vi "Show Hide (Label).vi"(5 "Invert? [F]":bool, 7 "Regex? [F]":bool, 8 "error in (no error)":errorcluster, 9 "Show? [T]":bool=TRUE, 10 "Label":string, 11 "MMI Scaling in":refnum<class "Alternative.lvclass">) -> (0 "error out":errorcluster, 2 "Match?":bool, 3 "MMI Scaling out":refnum<class "Alternative.lvclass">)   [LabVIEW 2021, in "Alternative.lvclass"]
doc: "Copyright 2018, Wiebe Walstra, wiebe@carya.nl."
uses:
  Alternative.lvclass
  C:/Projects/Dynamic-Scaling/Dynamic Scaling/IContainer/IContainer.lvclass
  IContainer.lvclass
  IObject.lvclass
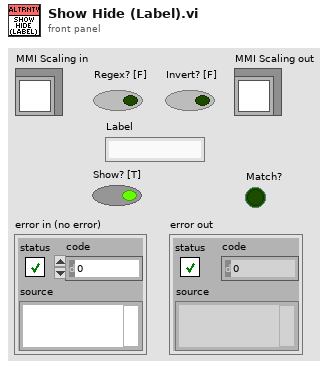
[diagram p1: front panel]
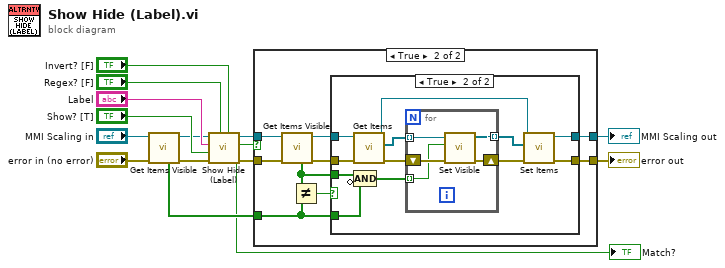
[diagram p0: block diagram]
diagram:
  n1 = call "Get Items Visible.vi"("error in (no error)"="error in (no error)", "IContainer in"="MMI Scaling in") -> ("error out"=w4:errorcluster, "IContainer out"=w7:refnum<class "Alternative.lvclass">, "Items visible"=w2:bool[])  [unwired: 6 in, 1 out]
  n2 = call-parent "Show Hide (Label).vi"("Invert? [F]"="Invert? [F]", "Regex? [F]"="Regex? [F]", "error in (no error)"=w4, "Show? [T]"="Show? [T]", "Label"="Label", "MMI Scaling in"=w7) -> ("error out"=w14:errorcluster, "Match?"=w1:bool, "MMI Scaling out"=w3:refnum<class "Alternative.lvclass">)  [unwired: 3 in]
  "Match?" <- w1
  n3 = case shown="True" w1 {
    tunnel: w14 -> [w15 w25]
    tunnel: [w15 w24] -> w9
    tunnel: [w16 w23] -> w8
    tunnel: w3 -> [w16 w21]
    tunnel: w2 -> [_ w18]
    frame False {
    }
    frame True {
      n4 = call "Get Items Visible.vi"("error in (no error)"=w25, "IContainer in"=w21) -> ("error out"=w22:errorcluster, "IContainer out"=w20:refnum<class "Alternative.lvclass">, "Items visible"=w19:bool[])  [unwired: 6 in, 1 out]
      n5 = Not Equal?(x=w19, y=w18) -> (x != y?=w17:bool)
      n6 = case shown="True" w17 {
        tunnel: w22 -> [w26 w39]
        tunnel: w20 -> [w27 w38]
        tunnel: [w26 w37] -> w24
        tunnel: [w27 w35] -> w23
        tunnel: w19 -> [_ w30]
        tunnel: w18 -> [_ w29]
        frame False {
        }
        frame True {
          n7 = call "Get Items.vi"("error in (no error)"=w39, "IContainer in"=w38) -> ("error out"=w32:errorcluster, "Items"=w34:refnum<class "IObject.lvclass">[], "IContainer out"=w36:refnum<class "Alternative.lvclass">)  [unwired: 7 in]
          n8 = Compound Arithmetic op=AND(w30, invert w29) -> (w28:bool[])
          n9 = for {
            tunnel: w34 -> [w42] mode=indexing
            shift-right: [w43] -> w33
            shift-left: w32 -> [w44]
            tunnel: [w41] -> w31 mode=indexing
            tunnel: w28 -> [w40] mode=indexing
            n10 = call-dynamic "Set Visible.vi"("error in (no error)"=w44, "Show? [T]"=w40, "MMI Scaling in"=w42) -> ("error out"=w43:errorcluster, "MMI Scaling out"=w41:refnum<class "IObject.lvclass">)  [unwired: 7 in]
          }
          n11 = call "Set Items.vi"("error in (no error)"=w33, "Items"=w31, "IContainer in"=w36) -> ("error out"=w37:errorcluster, "IContainer out"=w35:refnum<class "Alternative.lvclass">)  [unwired: 7 in]
        }
      }
    }
  }
  "error out" <- w9
  "MMI Scaling out" <- w8
